vi "New.vi"(7 "Parent":refnum<class "Abstract.lvclass">, 8 "Error In":errorcluster, 11 "Key":string) -> (0 "Error Out":errorcluster, 3 "Section":refnum<class "Section.lvclass">)   [LabVIEW 2018, in "Toolkit.lvlib" / "Nodes.lvlib" / "Section.lvclass"]
uses:
  Section.lvclass
  Abstract/Abstract.lvclass
  Section.lvclass/Section.ctl
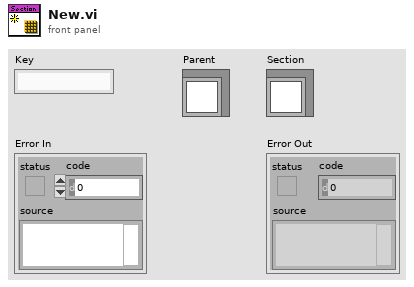
[diagram p1: front panel]
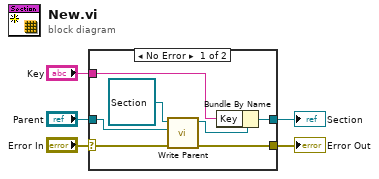
[diagram p0: block diagram]
diagram:
  n1 = case shown="No Error" "Error In" {
    selector: "Error In" -> [w9 w13]
    tunnel: "Parent" -> [w12 _]
    tunnel: [w10 w13] -> w4
    tunnel: [w7 _] -> w2
    tunnel: "Key" -> [w6 _]
    frame No Error {
      n2 = call-dynamic "Write Parent.vi"("Error In"=w9, "Parent"=w12, "Node In"=refnum<class "Section.lvclass"> refnum ("Toolkit.lvlib:Nodes.lvlib:Section.lvclass")) -> ("Error Out"=w10:errorcluster, "Node Out"=w8:refnum<class "Section.lvclass">)  [unwired: 7 in]
      n3 = Bundle By Name(cluster=w8, "Key"=w6) -> (w7:refnum<class "Section.lvclass">)
    }
    frame Error {
    }
  }
  "Error Out" <- w4
  "Section" <- w2
